vi "OR Error clusters.vi"(2 "error in 2":errorcluster, 3 "error in 1":errorcluster) -> (0 "error out 2":errorcluster, 1 "error out":errorcluster)   [LabVIEW 2013, in "Utility Lib.lvlib"]
doc: "This VI will OR the errors from two inputs. If either are true then it passes the true one out, if both are true it passes the error code from the first input and concatinates the second error into the source block. If both are false it passes the first error straight thru. Both of the output error clusters are wired together. This provides more flexibility in wiring the VI into the data flow."
uses:
  Utility Lib.lvlib
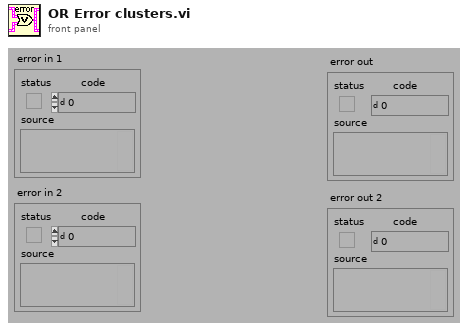
[diagram p1: front panel]
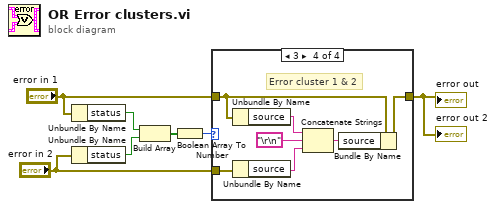
[diagram p0: block diagram]
diagram:
  n1 = Unbundle By Name("error in 1") -> ("status"=w7:bool)
  n2 = Unbundle By Name("error in 2") -> ("status"=w6:bool)
  n3 = Build Array(w7, w6) -> (w5:bool[])
  n4 = Boolean Array To Number(Boolean array=w5) -> (number=w4:u32)
  n5 = case shown="3" w4 {
    tunnel: "error in 1" -> [w8 w9 _ w12]
    tunnel: "error in 2" -> [_ _ w10 w17]
    tunnel: [w8 w9 w10 w11] -> w1
    frame 0, Default {
      # "No Errors"
    }
    frame 1 {
      # "Error Cluster 1"
    }
    frame 2 {
      # "Error Cluster 2"
    }
    frame 3 {
      # "Error cluster 1 & 2"
      n6 = Unbundle By Name(w12) -> ("source"=w16:string)
      n7 = Unbundle By Name(w17) -> ("source"=w15:string)
      n8 = Concatenate Strings(w16, "\r\n", w15) -> (w13:string)
      n9 = Bundle By Name(cluster=w12, "source"=w13) -> (w11:errorcluster)
    }
  }
  "error out" <- w1
  "error out 2" <- w1
